vi "Setup UI.vi"(8 "error in (no error)":errorcluster, 10 "Set UI to input? (F)":bool, 11 "Microwave Freq Scan in":refnum<class "Microwave Freq Scan.lvclass">) -> (0 "error out":errorcluster, 3 "Microwave Freq Scan out":refnum<class "Microwave Freq Scan.lvclass">)   [LabVIEW 2009, in "Microwave Freq Scan.lvclass"]
doc: "Scanner::Setup is a constructor that has no parameters and faces the user. The Factory calls this VI to let the user configure this Scanner. It is dynamically dispatched in order to let the user choose the type as well as the options of the scanner."
uses:
  Microwave Freq Scan.lvclass
  Microwave Freq Scan.lvclass/Microwave Freq Scan.ctl
panel:
  in  "Send conds for \nfirst point to MW Gen":bool
  in  "Amplitude (dBm)":dbl
  # "Microwave Freq Scan"
  # "Note: Independent variable \nabove must be given in GHz"
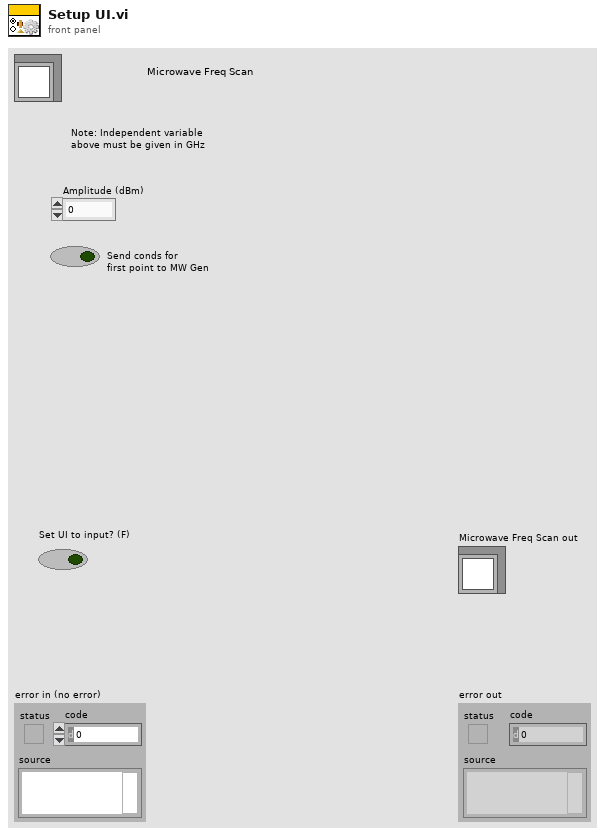
[diagram p1: front panel]
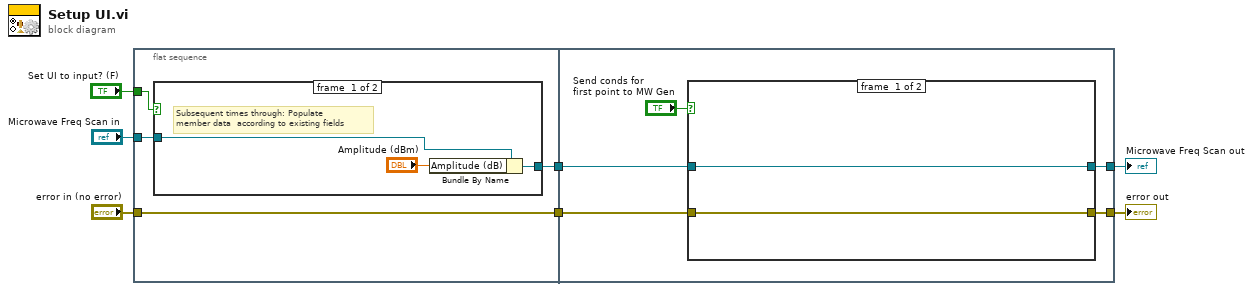
[diagram p0: block diagram]
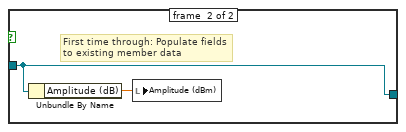
[diagram p2: hidden frame]
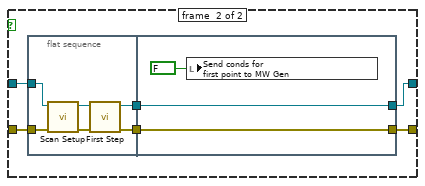
[diagram p3: hidden frame]
diagram:
  n1 = flat-sequence {
    tunnel: "Set UI to input? (F)" -> [w11]
    tunnel: [w10] -> w6
    tunnel: "Microwave Freq Scan in" -> [w9]
    tunnel: "error in (no error)" -> [w8]
    tunnel: [w8] -> w3
    tunnel: w6 -> [w20]
    tunnel: [w19] -> w5
    tunnel: [w18] -> w4
    tunnel: w3 -> [w17]
    frame #0 {
      n2 = case shown="True" w11 {
        tunnel: [w13 w16] -> w10
        tunnel: w9 -> [w14 w16]
        frame #0 {
          # "Subsequent times through: Populate \nmember data  according to existing fields"
          n3 = Bundle By Name(cluster=w14, "Amplitude (dB)"="Amplitude (dBm)") -> (w13:refnum<class "Microwave Freq Scan.lvclass">)
        }
        frame #1 {
          # "First time through: Populate fields  \nto existing member data"
          n4 = Unbundle By Name(w16) -> ("Amplitude (dB)"=w15:dbl)
          n5 = local write "Amplitude (dBm)"(w15) -> ()
        }
      }
    }
    frame #1 {
      n6 = case shown="True" "Send conds for \nfirst point to MW Gen" {
        tunnel: w20 -> [w23 w29]
        tunnel: [w23 w28] -> w19
        tunnel: [w22 w27] -> w18
        tunnel: w17 -> [w22 w26]
        frame #0 {
        }
        frame #1 {
          n7 = flat-sequence {
            tunnel: w29 -> [w33]
            tunnel: w26 -> [w30]
            tunnel: [w32] -> w25
            tunnel: [w31] -> w24
            tunnel: [w37] -> w27
            tunnel: [w38] -> w28
            tunnel: w25 -> [w38]
            tunnel: w24 -> [w37]
            frame #0 {
              n8 = call-dynamic "Scan Setup.vi"("error in (no error)"=w30, "Microwave Freq Scan in"=w33) -> ("error out"=w34:errorcluster, "Microwave Freq Scan out"=w35:refnum<class "Microwave Freq Scan.lvclass">)  [unwired: 8 out]
              n9 = call-dynamic "First Step.vi"("error in (no error)"=w34, "Microwave Freq Scan.lvclass in"=w35) -> ("error out"=w31:errorcluster, "Microwave Freq Scan.lvclass out"=w32:refnum<class "Microwave Freq Scan.lvclass">)  [unwired: 8 out]
            }
            frame #1 {
              n10 = local write "Send conds for \nfirst point to MW Gen"(FALSE ("Send conds for first point to MW Gen")) -> ()
            }
          }
        }
      }
    }
  }
  "error out" <- w4
  "Microwave Freq Scan out" <- w5
